vi "ps35demo.vi"() -> ()   [LabVIEW 2020]
uses:
  <vilib>/Utility/error.llb/DialogType.ctl
panel:
  in  "Index":i32
  out "JoyOn":bool
  out "axis3":i32
  out "axis2":i32
  out "axis1":i32
  out "Astat":string caption="Axis state string (123)"
  out "SpeedAct3":dbl caption="SpeedAct" format="%.3f"
  out "Target3":dbl caption="Target" format="%.3f"
  out "PosAct3":dbl caption="PosAct" format="%.3f"
  out "SpeedAct2":dbl caption="SpeedAct" format="%.3f"
  out "Target2":dbl caption="Target" format="%.3f"
  out "PosAct2":dbl caption="PosAct" format="%.3f"
  out "SpeedAct1":dbl caption="SpeedAct" format="%.3f"
  in  "PosMode3":u8(ring) caption="PosMode" items=["Trapeze", "S-curve"]
  in  "PosMode2":u8(ring) caption="PosMode" items=["Trapeze", "S-curve"]
  in  "TarMode3":u8(ring) caption="TarMode" items=["relative", "absolute"]
  in  "TarMode2":u8(ring) caption="TarMode" items=["relative", "absolute"]
  in  "TarMode1":u8(ring) caption="TarMode" items=["relative", "absolute"]
  in  "Go":bool
  in  "End":bool
  in  "Exit":bool
  in  "Stop3":bool
  in  "Motor3":bool
  in  "Stop2":bool
  in  "Motor2":bool
  in  "mm(deg)":bool
  in  "Inc":bool
  in  "Set tar":bool
  out "CheckOn":bool=TRUE
  in  "Stop1":bool
  in  "SwitchFree":bool
  out "Target1":dbl caption="Target" format="%.3f"
  out "PosAct1":dbl caption="PosAct" format="%.3f"
  in  "Set act":bool
  in  "Start":bool
  in  "Position, mm":dbl(knob) scale=-500.0..500.0 scale format="%.1f"
  in  "Position, Inc":i32(knob) scale=-1000000.0..1000000.0
  in  "PosMode1":u8(ring) caption="PosMode" items=["Trapeze", "S-curve"]
  in  "Number":i32=1 min=1 max=3
  in  "GoRef":bool
  in  "Motor1":bool
  # "Axis"
  # "Axis"
  # "Axis"
  # "Axis"
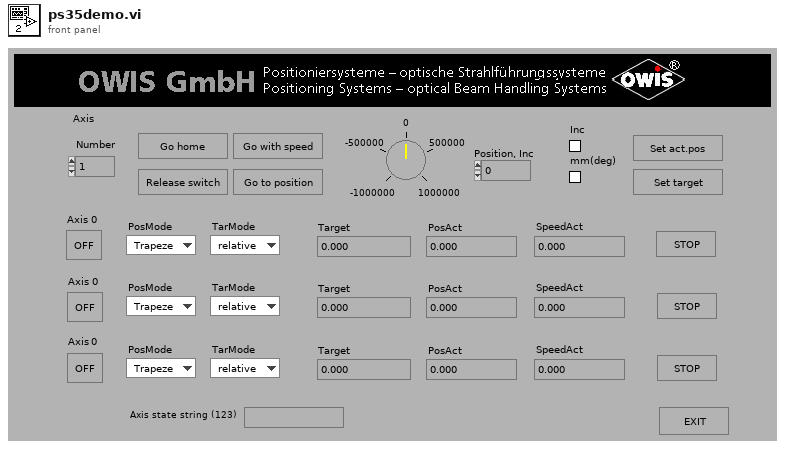
[diagram p1: front panel]
types:
  T1 = typedef "DialogType.ctl" = u16
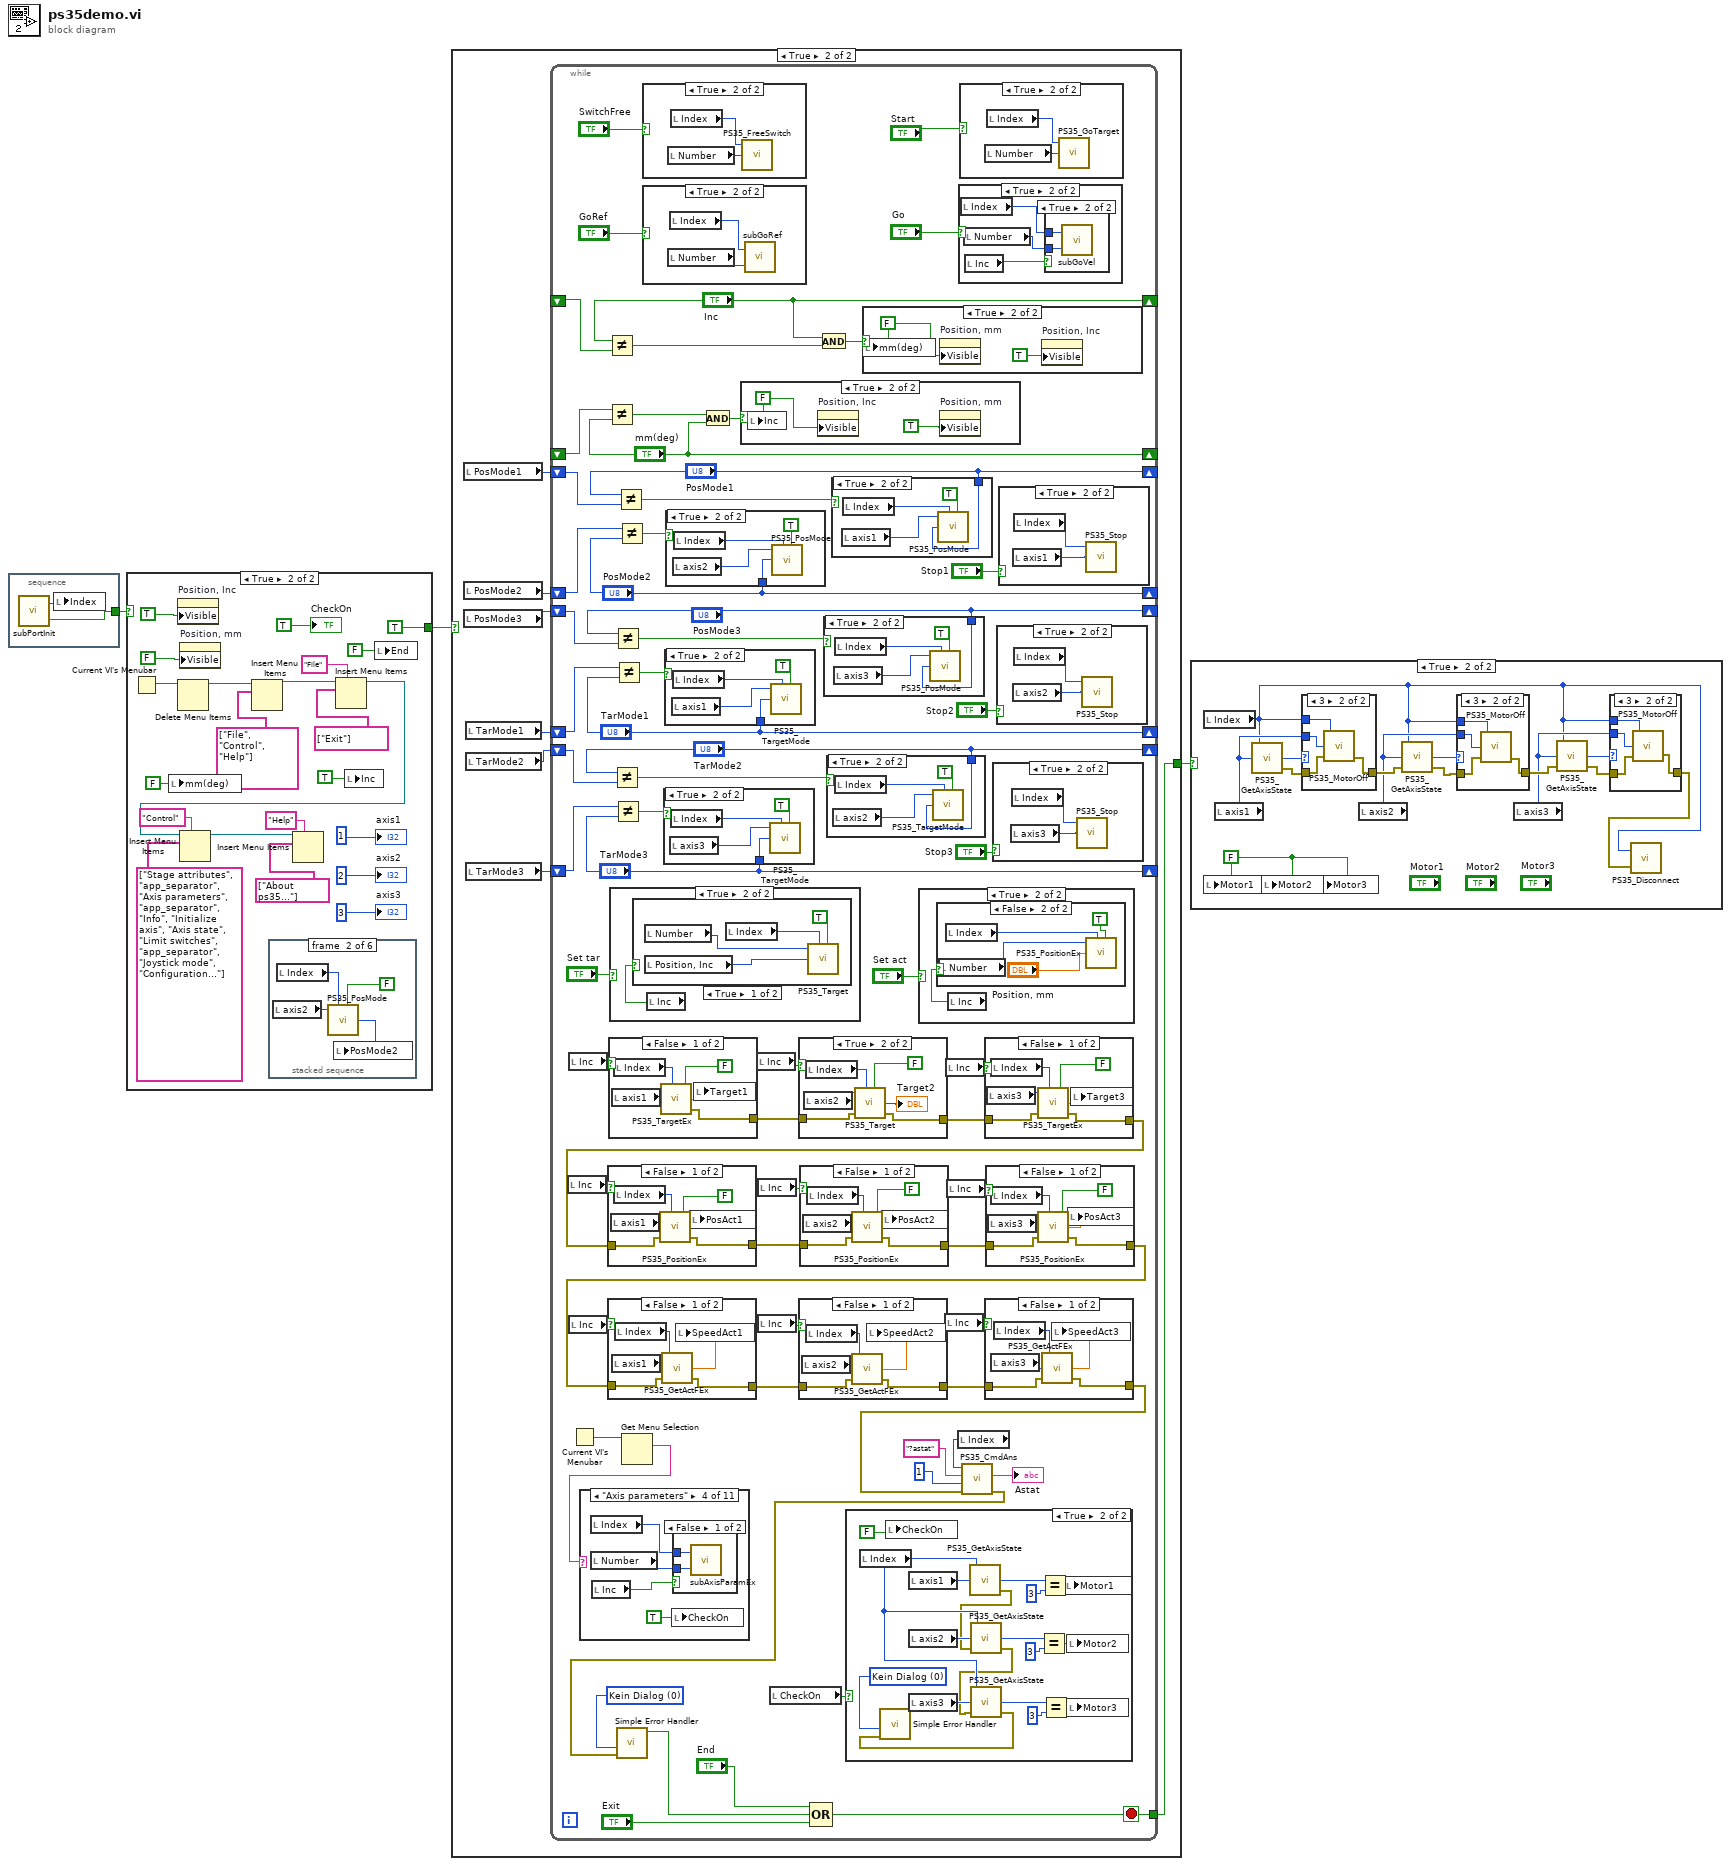
[diagram p0: block diagram]
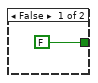
[diagram p2: hidden frame]
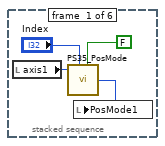
[diagram p3: hidden frame]
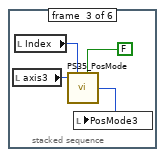
[diagram p4: hidden frame]
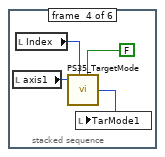
[diagram p5: hidden frame]
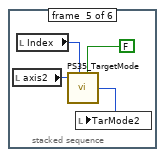
[diagram p6: hidden frame]
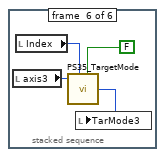
[diagram p7: hidden frame]
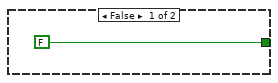
[diagram p12: hidden frame]
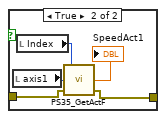
[diagram p13: hidden frame]
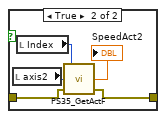
[diagram p14: hidden frame]
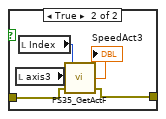
[diagram p15: hidden frame]
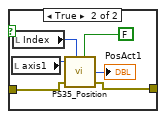
[diagram p16: hidden frame]
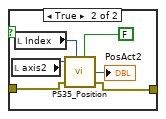
[diagram p17: hidden frame]
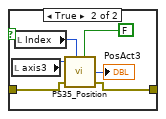
[diagram p18: hidden frame]
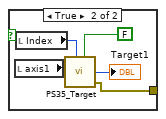
[diagram p19: hidden frame]
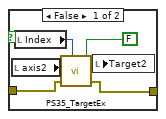
[diagram p20: hidden frame]
diagram:
  n1 = stacked-sequence {
    tunnel: [w5] -> w2
    frame #0 {
      n2 = call "subPortInit.vi"() -> ("Index"=w4:i32, "InitOK"=w5:bool)  [unwired: 1 in]
      n3 = local write "Index"(w4) -> ()
    }
  }
  n4 = case shown="True" w2 {
    tunnel: [FALSE TRUE] -> w1
    frame False {
    }
    frame True {
      n5 = Current VI's Menubar() -> (w21:refnum<k9>)
      n6 = local write "mm(deg)"(FALSE ("mm(deg)")) -> ()
      n7 = property on="Position, Inc" class="Knob (strict)"("Visible"=TRUE) -> ()  [unwired: 2 in, 2 out]
      n8 = Delete Menu Items(9:w21) -> (3:w22:refnum<k9>)  [unwired: 3 in, 1 out]
      n9 = property on="Position, mm" class="Knob (strict)"("Visible"=FALSE) -> ()  [unwired: 2 in, 2 out]
      n10 = Insert Menu Items(8:string[] ["File", "Control", "Help"], 9:w22) -> (3:w25:refnum<k9>)  [unwired: 4 in, 2 out]
      n11 = stacked-sequence {
        frame #0 {
          n12 = local read "axis1"() -> (w30:i32)
          n13 = call "PS35_PosMode.vi"("Axis number"=w30, "Control unit ID"="Index", "function"=FALSE ("WriteRead")) -> ("Value-Out"=w31:i32)  [unwired: 5 in, 1 out]
          n14 = local write "PosMode1"(w31) -> ()
        }
        frame #1 {
          n15 = local read "axis2"() -> (w34:i32)
          n16 = local read "Index"() -> (w33:i32)
          n17 = call "PS35_PosMode.vi"("Axis number"=w34, "Control unit ID"=w33, "function"=FALSE ("WriteRead")) -> ("Value-Out"=w35:i32)  [unwired: 5 in, 1 out]
          n18 = local write "PosMode2"(w35) -> ()
        }
        frame #2 {
          n19 = local read "axis3"() -> (w38:i32)
          n20 = local read "Index"() -> (w37:i32)
          n21 = call "PS35_PosMode.vi"("Axis number"=w38, "Control unit ID"=w37, "function"=FALSE ("WriteRead")) -> ("Value-Out"=w39:i32)  [unwired: 5 in, 1 out]
          n22 = local write "PosMode3"(w39) -> ()
        }
        frame #3 {
          n23 = local read "axis1"() -> (w42:i32)
          n24 = local read "Index"() -> (w41:i32)
          n25 = call "PS35_TargetMode.vi"("Axis number"=w42, "Control unit ID"=w41, "function"=FALSE ("WriteRead")) -> ("Value-Out"=w43:i32)  [unwired: 5 in, 1 out]
          n26 = local write "TarMode1"(w43) -> ()
        }
        frame #4 {
          n27 = local read "axis2"() -> (w46:i32)
          n28 = local read "Index"() -> (w45:i32)
          n29 = call "PS35_TargetMode.vi"("Axis number"=w46, "Control unit ID"=w45, "function"=FALSE ("WriteRead")) -> ("Value-Out"=w47:i32)  [unwired: 5 in, 1 out]
          n30 = local write "TarMode2"(w47) -> ()
        }
        frame #5 {
          n31 = local read "axis3"() -> (w50:i32)
          n32 = local read "Index"() -> (w49:i32)
          n33 = call "PS35_TargetMode.vi"("Axis number"=w50, "Control unit ID"=w49, "function"=FALSE ("WriteRead")) -> ("Value-Out"=w51:i32)  [unwired: 5 in, 1 out]
          n34 = local write "TarMode3"(w51) -> ()
        }
      }
      n35 = Insert Menu Items(5:"File" ("menu tag"), 8:string[] ["Exit"], 9:w25) -> (3:w18:refnum<k9>)  [unwired: 3 in, 2 out]
      n36 = Insert Menu Items(5:"Control" ("menu tag"), 8:string[] ["Stage attributes", "app_separator", "Axis parameters", "app_separator", "Info", "Initialize axis", "Axis state", "Limit switches", "app_separator", "Joystick mode", "Configuration..."], 9:w18) -> (3:w11:refnum<k9>)  [unwired: 3 in, 2 out]
      n37 = Insert Menu Items(5:"Help" ("menu tag"), 8:string[] ["About ps35..."], 9:w11) -> ()  [unwired: 3 in, 3 out]
      n38 = local write "Inc"(TRUE ("WriteRead")) -> ()
      n39 = local write "End"(FALSE ("stop? (T)")) -> ()
      "axis1" <- 1 ("axis1")
      "axis2" <- 2 ("axis3")
      "axis3" <- 3 ("axis3")
      "CheckOn" <- TRUE ("CheckOn")
    }
  }
  n40 = case shown="True" w1 {
    tunnel: [FALSE ("stop") w60] -> w3
    frame False {
    }
    frame True {
      n41 = local read "PosMode1"() -> (w59:u8)
      n42 = local read "PosMode2"() -> (w58:u8)
      n43 = local read "PosMode3"() -> (w57:u8)
      n44 = local read "TarMode1"() -> (w56:u8)
      n45 = local read "TarMode2"() -> (w55:u8)
      n46 = local read "TarMode3"() -> (w54:u8)
      n47 = while {
        shift-left: w54 -> [w93]
        shift-right: ["TarMode3"] -> _
        shift-left: w55 -> [w95]
        shift-right: ["TarMode2"] -> _
        shift-left: w56 -> [w100]
        shift-right: ["TarMode1"] -> _
        shift-left: w57 -> [w98]
        shift-right: ["PosMode3"] -> _
        shift-left: w58 -> [w104]
        shift-right: ["PosMode2"] -> _
        shift-left: _ -> [w116]
        shift-right: ["mm(deg)"] -> _
        shift-left: _ -> [w117]
        shift-right: ["Inc"] -> _
        tunnel: [w64] -> w60
        shift-left: w59 -> [w126]
        shift-right: ["PosMode1"] -> _
        stop <- w64 stop-if-true
        w63 = T1 0 items=["Kein Dialog", "OK-Nachricht", "Dialog zum Fortsetzen oder Anhalten", "OK Nachricht + Warnungen", "Weiter/Stop + Warnung"] ("type of dialog (OK msg:1)")
        n48 = local read "Inc"() -> (w80:bool)
        n49 = local read "Inc"() -> (w82:bool)
        n50 = local read "Inc"() -> (w77:bool)
        n51 = Current VI's Menubar() -> (w110:refnum<k9>)
        n52 = Not Equal?(x="Inc", y=w117) -> (x != y?=w118:bool)
        n53 = Not Equal?(x=w116, y="mm(deg)") -> (x != y?=w113:bool)
        n54 = case shown="False" w82 {
          tunnel: [w193 w198] -> w74
          frame False {
            n55 = local read "axis1"() -> (w197:i32)
            n56 = local read "Index"() -> (w194:i32)
            n57 = call "PS35_TargetEx.vi"("Axis number"=w197, "Control unit ID"=w194, "function"=FALSE ("WriteRead")) -> ("dValue-Out"=w196:dbl, "error out"=w193:errorcluster)  [unwired: 5 in]
            n58 = local write "Target1"(w196) -> ()
          }
          frame True {
            n59 = local read "axis1"() -> (w201:i32)
            n60 = local read "Index"() -> (w199:i32)
            n61 = call "PS35_Target.vi"("Axis number"=w201, "Control unit ID"=w199, "function"=FALSE ("WriteRead")) -> ("Value-Out"=→"Target1":i32, "error out"=w198:errorcluster)  [unwired: 5 in]
          }
        }
        n62 = case shown="True" "Set tar" {
          frame False {
          }
          frame True {
            n63 = local read "Inc"() -> (w316:bool)
            n64 = case shown="True" w316 {
              frame True {
                n65 = local read "Number"() -> (w320:i32)
                n66 = local read "Position, Inc"() -> (w319:i32)
                n67 = local read "Index"() -> (w317:i32)
                n68 = call "PS35_Target.vi"("Axis number"=w320, "Control unit ID"=w317, "Value-In"=w319, "function"=TRUE ("WriteRead")) -> ()  [unwired: 4 in, 2 out]
              }
              frame False {
                n69 = local read "Number"() -> (w324:i32)
                n70 = local read "Index"() -> (w321:i32)
                n71 = local read "Position, mm"() -> (w323:dbl)
                n72 = call "PS35_TargetEx.vi"("Axis number"=w324, "Control unit ID"=w321, "dValue-In"=w323, "function"=TRUE ("WriteRead")) -> ()  [unwired: 4 in, 2 out]
              }
            }
          }
        }
        n73 = Not Equal?(x="TarMode2", y=w95) -> (x != y?=w94:bool)
        n74 = Not Equal?(x="PosMode3", y=w98) -> (x != y?=w99:bool)
        n75 = Not Equal?(x=w93, y="TarMode3") -> (x != y?=w92:bool)
        n76 = Not Equal?(x=w100, y="TarMode1") -> (x != y?=w101:bool)
        n77 = Not Equal?(x="PosMode1", y=w126) -> (x != y?=w125:bool)
        n78 = Not Equal?(x=w104, y="PosMode2") -> (x != y?=w103:bool)
        n79 = Get Menu Selection(0:w110) -> (6:w109:string)  [unwired: 3 in, 4 out]
        n80 = case shown="\"Axis parameters\"" w109 {
          frame "", Default {
          }
          frame "Exit" {
            n81 = local write "End"(TRUE ("stop? (T)")) -> ()
          }
          frame "Stage attributes" {
            n82 = local read "Number"() -> (w283:i32)
            n83 = local read "Index"() -> (w281:i32)
            n84 = local write "CheckOn"(TRUE ("CheckOn")) -> ()
            n85 = call "subSetStage.vi"("AxisId"=w283, "Index"=w281) -> ()  [unwired: 1 in]
          }
          frame "Axis parameters" {
            n86 = local read "Index"() -> (w285:i32)
            n87 = local read "Number"() -> (w287:i32)
            n88 = local read "Inc"() -> (w284:bool)
            n89 = local write "CheckOn"(TRUE ("CheckOn")) -> ()
            n90 = case shown="False" w284 {
              tunnel: w287 -> [w289 w291]
              tunnel: w285 -> [w288 w290]
              frame False {
                n91 = call "subAxisParamEx.vi"("AxisId"=w289, "Index"=w288) -> ()  [unwired: 1 in]
              }
              frame True {
                n92 = call "subAxisParam.vi"("AxisId"=w291, "Index"=w290) -> ()  [unwired: 1 in]
              }
            }
          }
          frame "Info" {
            n93 = local read "Index"() -> (w292:i32)
            n94 = local write "CheckOn"(TRUE ("CheckOn")) -> ()
            n95 = call "subFirmware.vi"("Index"=w292) -> ()  [unwired: 1 in]
          }
          frame "Initialize axis" {
            n96 = local read "Index"() -> (w294:i32)
            n97 = local read "Number"() -> (w296:i32)
            n98 = local write "CheckOn"(TRUE ("CheckOn")) -> ()
            n99 = call "PS35_MotorInit.vi"("Axis number"=w296, "Control unit ID"=w294) -> ()  [unwired: 2 in, 1 out]
          }
          frame "Axis state" {
            n100 = local read "Number"() -> (w299:i32)
            n101 = local read "Index"() -> (w297:i32)
            n102 = local write "CheckOn"(TRUE ("CheckOn")) -> ()
            n103 = call "subAxisState.vi"("AxisId"=w299, "Index"=w297) -> ()  [unwired: 1 in]
          }
          frame "Limit switches" {
            n104 = local read "Number"() -> (w302:i32)
            n105 = local read "Index"() -> (w300:i32)
            n106 = local write "CheckOn"(TRUE ("CheckOn")) -> ()
            n107 = call "subSwitches.vi"("AxisId"=w302, "Index"=w300) -> ()  [unwired: 1 in]
          }
          frame "Joystick mode" {
            n108 = local read "JoyOn"() -> (w303:bool)
            n109 = case shown="False" w303 {
              frame False {
                n110 = local read "Index"() -> (w304:i32)
                n111 = call "PS35_JoystickOn.vi"("Control unit ID"=w304) -> ()  [unwired: 2 in, 1 out]
                "JoyOn" <- TRUE ("JoyOn")
              }
              frame True {
                n112 = local read "Index"() -> (w306:i32)
                n113 = local write "JoyOn"(FALSE ("JoyOn")) -> ()
                n114 = call "PS35_JoystickOff.vi"("Control unit ID"=w306) -> ()  [unwired: 2 in, 1 out]
              }
            }
          }
          frame "Configuration..." {
            n115 = local read "Index"() -> (w309:i32)
            n116 = local read "Inc"() -> (w308:bool)
            n117 = case shown="True" w308 {
              tunnel: w309 -> [w310 w311]
              frame False {
                n118 = call "subJoystickEx.vi"("Index"=w310) -> ()  [unwired: 1 in]
              }
              frame True {
                n119 = call "subJoystick.vi"("Index"=w311) -> ()  [unwired: 1 in]
              }
            }
          }
          frame "About ps35..." {
            n120 = call "subSoftinfo.vi"() -> ()  [unwired: 1 in]
          }
        }
        n121 = case shown="True" "SwitchFree" {
          frame False {
          }
          frame True {
            n122 = local read "Number"() -> (w272:i32)
            n123 = local read "Index"() -> (w271:i32)
            n124 = call "PS35_FreeSwitch.vi"("Axis number"=w272, "Control unit ID"=w271) -> ()  [unwired: 2 in, 1 out]
          }
        }
        n125 = case shown="True" "GoRef" {
          frame False {
          }
          frame True {
            n126 = local read "Number"() -> (w270:i32)
            n127 = local read "Index"() -> (w269:i32)
            n128 = call "subGoRef.vi"("AxisId"=w270, "Index"=w269) -> ()  [unwired: 1 in]
          }
        }
        n129 = case shown="True" w92 {
          tunnel: "TarMode3" -> [_ w250]
          frame False {
          }
          frame True {
            n130 = local read "axis3"() -> (w251:i32)
            n131 = local read "Index"() -> (w249:i32)
            n132 = call "PS35_TargetMode.vi"("Axis number"=w251, "Control unit ID"=w249, "Value-In"=w250, "function"=TRUE ("WriteRead")) -> ()  [unwired: 4 in, 2 out]
          }
        }
        n133 = case shown="True" w101 {
          tunnel: "TarMode1" -> [_ w262]
          frame False {
          }
          frame True {
            n134 = local read "axis1"() -> (w263:i32)
            n135 = local read "Index"() -> (w261:i32)
            n136 = call "PS35_TargetMode.vi"("Axis number"=w263, "Control unit ID"=w261, "Value-In"=w262, "function"=TRUE ("WriteRead")) -> ()  [unwired: 4 in, 2 out]
          }
        }
        n137 = case shown="True" w103 {
          tunnel: "PosMode2" -> [_ w266]
          frame False {
          }
          frame True {
            n138 = local read "axis2"() -> (w267:i32)
            n139 = local read "Index"() -> (w265:i32)
            n140 = call "PS35_PosMode.vi"("Axis number"=w267, "Control unit ID"=w265, "Value-In"=w266, "function"=TRUE ("WriteRead")) -> ()  [unwired: 4 in, 2 out]
          }
        }
        n141 = And(x=w113, y="mm(deg)") -> (x .and. y?=w111:bool)
        n142 = case shown="True" w111 {
          frame False {
          }
          frame True {
            w312 = FALSE ("WriteRead")
            n143 = local write "Inc"(w312) -> ()
            n144 = property on="Position, Inc" class="Knob (strict)"("Visible"=w312) -> ()  [unwired: 2 in, 2 out]
            n145 = property on="Position, mm" class="Knob (strict)"("Visible"=TRUE) -> ()  [unwired: 2 in, 2 out]
          }
        }
        n146 = local read "Inc"() -> (w81:bool)
        n147 = local read "Inc"() -> (w79:bool)
        n148 = local read "Inc"() -> (w76:bool)
        n149 = local read "CheckOn"() -> (w84:bool)
        n150 = case shown="True" w81 {
          tunnel: w74 -> [w204 w210]
          tunnel: [w203 w209] -> w73
          frame False {
            n151 = local read "axis2"() -> (w208:i32)
            n152 = local read "Index"() -> (w205:i32)
            n153 = call "PS35_TargetEx.vi"("Axis number"=w208, "Control unit ID"=w205, "error in (no error)"=w204, "function"=FALSE ("WriteRead")) -> ("dValue-Out"=w207:dbl, "error out"=w203:errorcluster)  [unwired: 4 in]
            n154 = local write "Target2"(w207) -> ()
          }
          frame True {
            n155 = local read "axis2"() -> (w213:i32)
            n156 = local read "Index"() -> (w211:i32)
            n157 = call "PS35_Target.vi"("Axis number"=w213, "Control unit ID"=w211, "error in (no error)"=w210, "function"=FALSE ("WriteRead")) -> ("Value-Out"=→"Target2":i32, "error out"=w209:errorcluster)  [unwired: 4 in]
          }
        }
        n158 = And(x="Inc", y=w118) -> (x .and. y?=w115:bool)
        n159 = case shown="True" w99 {
          tunnel: "PosMode3" -> [_ w260]
          frame False {
          }
          frame True {
            n160 = local read "axis3"() -> (w258:i32)
            n161 = local read "Index"() -> (w257:i32)
            n162 = call "PS35_PosMode.vi"("Axis number"=w258, "Control unit ID"=w257, "Value-In"=w260, "function"=TRUE ("WriteRead")) -> ()  [unwired: 4 in, 2 out]
          }
        }
        n163 = case shown="True" w94 {
          tunnel: "TarMode2" -> [_ w256]
          frame False {
          }
          frame True {
            n164 = local read "axis2"() -> (w254:i32)
            n165 = local read "Index"() -> (w253:i32)
            n166 = call "PS35_TargetMode.vi"("Axis number"=w254, "Control unit ID"=w253, "Value-In"=w256, "function"=TRUE ("WriteRead")) -> ()  [unwired: 4 in, 2 out]
          }
        }
        n167 = case shown="True" w125 {
          tunnel: "PosMode1" -> [_ w341]
          frame False {
          }
          frame True {
            n168 = local read "axis1"() -> (w339:i32)
            n169 = local read "Index"() -> (w338:i32)
            n170 = call "PS35_PosMode.vi"("Axis number"=w339, "Control unit ID"=w338, "Value-In"=w341, "function"=TRUE ("WriteRead")) -> ()  [unwired: 4 in, 2 out]
          }
        }
        n171 = case shown="True" w84 {
          frame False {
          }
          frame True {
            w227 = T1 0 items=["Kein Dialog", "OK-Nachricht", "Dialog zum Fortsetzen oder Anhalten", "OK Nachricht + Warnungen", "Weiter/Stop + Warnung"] ("type of dialog (OK msg:1)")
            n172 = local read "Index"() -> (w231:i32)
            n173 = local write "CheckOn"(FALSE ("CheckOn")) -> ()
            n174 = local read "axis1"() -> (w235:i32)
            n175 = local read "axis2"() -> (w241:i32)
            n176 = local read "axis3"() -> (w240:i32)
            n177 = call "PS35_GetAxisState.vi"("Axis number"=w235, "Control unit ID"=w231) -> ("error out"=w230:errorcluster, "Axis state"=w234:i32)  [unwired: 2 in]
            n178 = call "PS35_GetAxisState.vi"("error in (no error)"=w230, "Axis number"=w241, "Control unit ID"=w231) -> ("error out"=w229:errorcluster, "Axis state"=w242:i32)  [unwired: 1 in]
            n179 = call "PS35_GetAxisState.vi"("error in (no error)"=w229, "Axis number"=w240, "Control unit ID"=w231) -> ("error out"=w228:errorcluster, "Axis state"=w239:i32)  [unwired: 1 in]
            n180 = call <vilib>:"Simple Error Handler.vi"("type of dialog (OK msg:1)"=w227, "error in (no error)"=w228) -> ()  [unwired: 3 in, 5 out]
            n181 = Equal?(x=w242, y=3) -> (x = y?=w244:bool)
            n182 = Equal?(x=w234, y=3) -> (x = y?=w232:bool)
            n183 = Equal?(x=w239, y=3) -> (x = y?=w237:bool)
            n184 = local write "Motor1"(w232) -> ()
            n185 = local write "Motor2"(w244) -> ()
            n186 = local write "Motor3"(w237) -> ()
          }
        }
        n187 = case shown="True" w115 {
          frame False {
          }
          frame True {
            w314 = FALSE ("WriteRead")
            n188 = local write "mm(deg)"(w314) -> ()
            n189 = property on="Position, mm" class="Knob (strict)"("Visible"=w314) -> ()  [unwired: 2 in, 2 out]
            n190 = property on="Position, Inc" class="Knob (strict)"("Visible"=TRUE) -> ()  [unwired: 2 in, 2 out]
          }
        }
        n191 = case shown="True" "Set act" {
          frame False {
          }
          frame True {
            n192 = local read "Inc"() -> (w329:bool)
            n193 = case shown="False" w329 {
              frame True {
                n194 = local read "Index"() -> (w330:i32)
                n195 = call "PS35_Position.vi"("Axis number"="Number", "Control unit ID"=w330, "Value-In"="Position, Inc", "function"=TRUE ("WriteRead")) -> ()  [unwired: 4 in, 2 out]
              }
              frame False {
                n196 = local read "Number"() -> (w337:i32)
                n197 = local read "Index"() -> (w334:i32)
                n198 = call "PS35_PositionEx.vi"("Axis number"=w337, "Control unit ID"=w334, "dValue-In"="Position, mm", "function"=TRUE ("WriteRead")) -> ()  [unwired: 4 in, 2 out]
              }
            }
          }
        }
        n199 = local read "Inc"() -> (w75:bool)
        n200 = local read "Inc"() -> (w83:bool)
        n201 = local read "Inc"() -> (w78:bool)
        n202 = local read "Index"() -> (w66:i32)
        n203 = case shown="True" "Go" {
          frame False {
          }
          frame True {
            n204 = local read "Index"() -> (w274:i32)
            n205 = local read "Number"() -> (w275:i32)
            n206 = local read "Inc"() -> (w273:bool)
            n207 = case shown="True" w273 {
              tunnel: w275 -> [w277 w279]
              tunnel: w274 -> [w276 w278]
              frame False {
                n208 = call "subGoVelEx.vi"("AxisId"=w277, "Index"=w276) -> ()  [unwired: 1 in]
              }
              frame True {
                n209 = call "subGoVel.vi"("AxisId"=w279, "Index"=w278) -> ()  [unwired: 1 in]
              }
            }
          }
        }
        n210 = case shown="True" "Start" {
          frame False {
          }
          frame True {
            n211 = local read "Number"() -> (w328:i32)
            n212 = local read "Index"() -> (w327:i32)
            n213 = call "PS35_GoTarget.vi"("Axis number"=w328, "Control unit ID"=w327) -> ()  [unwired: 2 in, 1 out]
          }
        }
        n214 = case shown="False" w83 {
          tunnel: w73 -> [w216 w222]
          tunnel: [w215 w221] -> w72
          frame False {
            n215 = local read "axis3"() -> (w220:i32)
            n216 = local read "Index"() -> (w217:i32)
            n217 = call "PS35_TargetEx.vi"("Axis number"=w220, "Control unit ID"=w217, "error in (no error)"=w216, "function"=FALSE ("WriteRead")) -> ("dValue-Out"=w219:dbl, "error out"=w215:errorcluster)  [unwired: 4 in]
            n218 = local write "Target3"(w219) -> ()
          }
          frame True {
            n219 = local read "axis3"() -> (w225:i32)
            n220 = local read "Index"() -> (w223:i32)
            n221 = call "PS35_Target.vi"("Axis number"=w225, "Control unit ID"=w223, "error in (no error)"=w222, "function"=FALSE ("WriteRead")) -> ("Value-Out"=→"Target3":i32, "error out"=w221:errorcluster)  [unwired: 4 in]
          }
        }
        n222 = case shown="False" w80 {
          tunnel: w72 -> [w158 w164]
          tunnel: [w157 w163] -> w71
          frame False {
            n223 = local read "axis1"() -> (w162:i32)
            n224 = local read "Index"() -> (w159:i32)
            n225 = call "PS35_PositionEx.vi"("Axis number"=w162, "Control unit ID"=w159, "error in (no error)"=w158, "function"=FALSE ("WriteRead")) -> ("dValue-Out"=w161:dbl, "error out"=w157:errorcluster)  [unwired: 4 in]
            n226 = local write "PosAct1"(w161) -> ()
          }
          frame True {
            n227 = local read "axis1"() -> (w167:i32)
            n228 = local read "Index"() -> (w165:i32)
            n229 = call "PS35_Position.vi"("Axis number"=w167, "Control unit ID"=w165, "error in (no error)"=w164, "function"=FALSE ("WriteRead")) -> ("Value-Out"=→"PosAct1":i32, "error out"=w163:errorcluster)  [unwired: 4 in]
          }
        }
        n230 = case shown="False" w79 {
          tunnel: w71 -> [w170 w176]
          tunnel: [w169 w175] -> w70
          frame False {
            n231 = local read "axis2"() -> (w174:i32)
            n232 = local read "Index"() -> (w171:i32)
            n233 = call "PS35_PositionEx.vi"("Axis number"=w174, "Control unit ID"=w171, "error in (no error)"=w170, "function"=FALSE ("WriteRead")) -> ("dValue-Out"=w173:dbl, "error out"=w169:errorcluster)  [unwired: 4 in]
            n234 = local write "PosAct2"(w173) -> ()
          }
          frame True {
            n235 = local read "axis2"() -> (w179:i32)
            n236 = local read "Index"() -> (w177:i32)
            n237 = call "PS35_Position.vi"("Axis number"=w179, "Control unit ID"=w177, "error in (no error)"=w176, "function"=FALSE ("WriteRead")) -> ("Value-Out"=→"PosAct2":i32, "error out"=w175:errorcluster)  [unwired: 4 in]
          }
        }
        n238 = case shown="False" w78 {
          tunnel: w70 -> [w182 w188]
          tunnel: [w181 w187] -> w69
          frame False {
            n239 = local read "axis3"() -> (w186:i32)
            n240 = local read "Index"() -> (w183:i32)
            n241 = call "PS35_PositionEx.vi"("Axis number"=w186, "Control unit ID"=w183, "error in (no error)"=w182, "function"=FALSE ("WriteRead")) -> ("dValue-Out"=w185:dbl, "error out"=w181:errorcluster)  [unwired: 4 in]
            n242 = local write "PosAct3"(w185) -> ()
          }
          frame True {
            n243 = local read "axis3"() -> (w191:i32)
            n244 = local read "Index"() -> (w189:i32)
            n245 = call "PS35_Position.vi"("Axis number"=w191, "Control unit ID"=w189, "error in (no error)"=w188, "function"=FALSE ("WriteRead")) -> ("Value-Out"=→"PosAct3":i32, "error out"=w187:errorcluster)  [unwired: 4 in]
          }
        }
        n246 = case shown="False" w77 {
          tunnel: w69 -> [w128 w133]
          tunnel: [w127 w132] -> w68
          frame False {
            n247 = local read "axis1"() -> (w131:i32)
            n248 = local read "Index"() -> (w129:i32)
            n249 = call "PS35_GetActFEx.vi"("error in (no error)"=w128, "Axis number"=w131, "Control unit ID"=w129) -> ("error out"=w127:errorcluster, "dValue"=w130:dbl)  [unwired: 1 in]
            n250 = local write "SpeedAct1"(w130) -> ()
          }
          frame True {
            n251 = local read "axis1"() -> (w136:i32)
            n252 = local read "Index"() -> (w134:i32)
            n253 = call "PS35_GetActF.vi"("error in (no error)"=w133, "Axis number"=w136, "Control unit ID"=w134) -> ("error out"=w132:errorcluster, "dValue"=→"SpeedAct1":dbl)  [unwired: 1 in]
          }
        }
        n254 = case shown="False" w76 {
          tunnel: w68 -> [w138 w143]
          tunnel: [w137 w142] -> w67
          frame False {
            n255 = local read "axis2"() -> (w141:i32)
            n256 = local read "Index"() -> (w139:i32)
            n257 = call "PS35_GetActFEx.vi"("error in (no error)"=w138, "Axis number"=w141, "Control unit ID"=w139) -> ("error out"=w137:errorcluster, "dValue"=w140:dbl)  [unwired: 1 in]
            n258 = local write "SpeedAct2"(w140) -> ()
          }
          frame True {
            n259 = local read "axis2"() -> (w146:i32)
            n260 = local read "Index"() -> (w144:i32)
            n261 = call "PS35_GetActF.vi"("error in (no error)"=w143, "Axis number"=w146, "Control unit ID"=w144) -> ("error out"=w142:errorcluster, "dValue"=→"SpeedAct2":dbl)  [unwired: 1 in]
          }
        }
        n262 = case shown="False" w75 {
          tunnel: w67 -> [w148 w153]
          tunnel: [w147 w152] -> w65
          frame False {
            n263 = local read "axis3"() -> (w151:i32)
            n264 = local read "Index"() -> (w149:i32)
            n265 = call "PS35_GetActFEx.vi"("error in (no error)"=w148, "Axis number"=w151, "Control unit ID"=w149) -> ("error out"=w147:errorcluster, "dValue"=w150:dbl)  [unwired: 1 in]
            n266 = local write "SpeedAct3"(w150) -> ()
          }
          frame True {
            n267 = local read "axis3"() -> (w156:i32)
            n268 = local read "Index"() -> (w154:i32)
            n269 = call "PS35_GetActF.vi"("error in (no error)"=w153, "Axis number"=w156, "Control unit ID"=w154) -> ("error out"=w152:errorcluster, "dValue"=→"SpeedAct3":dbl)  [unwired: 1 in]
          }
        }
        n270 = call "PS35_CmdAns.vi"("error in (no error)"=w65, "nRequest"=u8 1 ("bRequest"), "Command"="?astat", "Control unit ID"=w66) -> ("error out"=w62:errorcluster, "Answer string"=→"Astat":string)  [unwired: 1 in, 1 out]
        n271 = call <vilib>:"Simple Error Handler.vi"("type of dialog (OK msg:1)"=w63, "error in (no error)"=w62) -> ("error?"=w61:bool)  [unwired: 3 in, 4 out]
        n272 = Compound Arithmetic op=OR("End", w61, "Exit") -> (w64:bool)
        n273 = case shown="True" "Stop3" {
          frame False {
          }
          frame True {
            n274 = local read "axis3"() -> (w246:i32)
            n275 = local read "Index"() -> (w245:i32)
            n276 = call "PS35_Stop.vi"("Axis number"=w246, "Control unit ID"=w245) -> ()  [unwired: 2 in, 1 out]
          }
        }
        n277 = case shown="True" "Stop2" {
          frame False {
          }
          frame True {
            n278 = local read "axis2"() -> (w248:i32)
            n279 = local read "Index"() -> (w247:i32)
            n280 = call "PS35_Stop.vi"("Axis number"=w248, "Control unit ID"=w247) -> ()  [unwired: 2 in, 1 out]
          }
        }
        n281 = case shown="True" "Stop1" {
          frame False {
          }
          frame True {
            n282 = local read "axis1"() -> (w326:i32)
            n283 = local read "Index"() -> (w325:i32)
            n284 = call "PS35_Stop.vi"("Axis number"=w326, "Control unit ID"=w325) -> ()  [unwired: 2 in, 1 out]
          }
        }
      }
    }
  }
  n285 = case shown="True" w3 {
    frame False {
    }
    frame True {
      w354 = FALSE ("WriteRead")
      n286 = local read "Index"() -> (w342:i32)
      n287 = local write "Motor1"(w354) -> ()
      n288 = local read "axis1"() -> (w353:i32)
      n289 = call "PS35_GetAxisState.vi"("Axis number"=w353, "Control unit ID"=w342) -> ("error out"=w352:errorcluster, "Axis state"=w355:i32)  [unwired: 2 in]
      n290 = local write "Motor2"(w354) -> ()
      n291 = case shown="3" w355 {
        tunnel: w342 -> [_ w370]
        tunnel: w353 -> [_ w369]
        tunnel: w352 -> [w366 w368]
        tunnel: [w366 w367] -> w351
        frame 0, Default {
        }
        frame 3 {
          n292 = call "PS35_MotorOff.vi"("error in (no error)"=w368, "Axis number"=w369, "Control unit ID"=w370) -> ("error out"=w367:errorcluster)  [unwired: 1 in]
        }
      }
      n293 = local write "Motor3"(w354) -> ()
      n294 = local read "axis2"() -> (w348:i32)
      n295 = call "PS35_GetAxisState.vi"("error in (no error)"=w351, "Axis number"=w348, "Control unit ID"=w342) -> ("error out"=w349:errorcluster, "Axis state"=w350:i32)  [unwired: 1 in]
      n296 = case shown="3" w350 {
        tunnel: w342 -> [_ w365]
        tunnel: w349 -> [w361 w364]
        tunnel: [w361 w363] -> w346
        tunnel: w348 -> [_ w362]
        frame 0, Default {
        }
        frame 3 {
          n297 = call "PS35_MotorOff.vi"("error in (no error)"=w364, "Axis number"=w362, "Control unit ID"=w365) -> ("error out"=w363:errorcluster)  [unwired: 1 in]
        }
      }
      n298 = local read "axis3"() -> (w343:i32)
      n299 = call "PS35_GetAxisState.vi"("error in (no error)"=w346, "Axis number"=w343, "Control unit ID"=w342) -> ("error out"=w345:errorcluster, "Axis state"=w347:i32)  [unwired: 1 in]
      n300 = case shown="3" w347 {
        tunnel: w345 -> [w356 w360]
        tunnel: [w356 w359] -> w344
        tunnel: w342 -> [_ w358]
        tunnel: w343 -> [_ w357]
        frame 0, Default {
        }
        frame 3 {
          n301 = call "PS35_MotorOff.vi"("error in (no error)"=w360, "Axis number"=w357, "Control unit ID"=w358) -> ("error out"=w359:errorcluster)  [unwired: 1 in]
        }
      }
      n302 = call "PS35_Disconnect.vi"("error in (no error)"=w344, "Control unit ID"=w342) -> ()  [unwired: 1 in, 1 out]
    }
  }
